vi "strict.Assert To Report Entry.vi"(8 "error in (no error)":errorcluster, 10 "Assert":T1={"Name"="", "Passed"=FALSE, "Call Chain"=[], "Test Error"={"status"=FALSE, "code"=0, "source"=""}, "Time Stamp"=timestamp(0 s since 1904-01-01), "Unique Assert ID"="", "Test ID"="", "Execution time (s)"=-1.0, "Verbose Explanation"=""}) -> (0 "error out":errorcluster, 2 "String":string)   [LabVIEW 2013, in "strict-JUnit.lvclass"]
uses:
  strict-JUnit.lvclass
  <vilib>/addons/_JKI Toolkits/Caraya/classes/Test Result/Assert Event Data.ctl
  <vilib>/addons/_JKI Toolkits/Caraya/classes/Test Report/Test Report.lvclass
  <vilib>/addons/_JKI Toolkits/Caraya/classes/Test Result/Test Result.lvclass
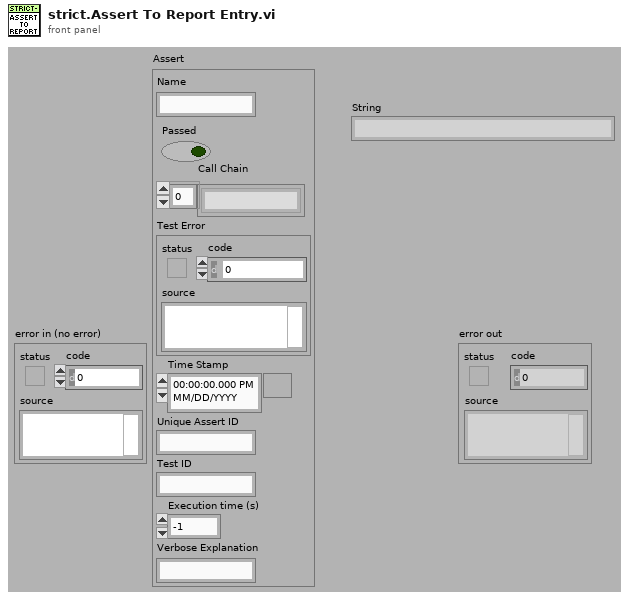
[diagram p1: front panel]
types:
  T1 = typedef "Caraya.lvlib/Test Result.lvclass/Assert Event Data.ctl" = cluster{"Name":string, "Passed":bool, "Call Chain":string[], "Test Error":errorcluster, "Time Stamp":timestamp, "Unique Assert ID":string, "Test ID":string, "Execution time (s)":dbl, "Verbose Explanation":string}
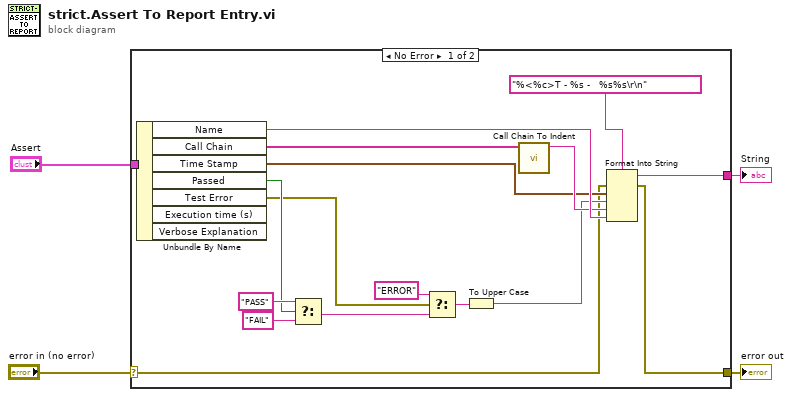
[diagram p0: block diagram]
diagram:
  n1 = case shown="No Error" "error in (no error)" {
    selector: "error in (no error)" -> [w9 w22]
    tunnel: [w19 w22] -> w3
    tunnel: "Assert" -> [w16 _]
    tunnel: [w18 _] -> w1
    frame No Error {
      n2 = Unbundle By Name(w16) -> ("Name"=w20:string, "Call Chain"=w15:string[], "Time Stamp"=w14:timestamp, "Passed"=w6:bool, "Test Error"=w5:errorcluster)  [unwired: 2 out]
      n3 = Select(t="PASS" ("format string"), s=w6, f="FAIL" ("format string")) -> (s? t:f=w8:string)
      n4 = Select(t="ERROR" ("format string"), s=w5, f=w8) -> (s? t:f=w11:string)
      n5 = To Upper Case(1:w11) -> (0:w10:string)
      n6 = call <vilib>:"Call Chain To Indent.vi"("Call Chain"=w15) -> ("Indent"=w17:string)  [unwired: 10 in]
      n7 = Format Into String(format string="%<%c>T - %s -   %s%s\r\n", error in=w9, w14, w10, w17, w20) -> (resulting string=w18:string, error out=w19:errorcluster)  [unwired: 1 in]
    }
    frame Error {
    }
  }
  "error out" <- w3
  "String" <- w1
